vi "solar_cfg Simple.vi"(4 "Write If Not Found? (T)":bool=TRUE, 5 "Action (Read)":enum8{"Read", "Write"}(ring), 6 "Replace Existing Comments? (F)":bool, 7 "Section (\"\" = Filename)":string, 8 "error in (no error)":errorcluster, 10 "Key,Value,Comment":string[][](array[string]), 11 "Config Path (*.ini)":path) -> (0 "error out":errorcluster, 1 "Found?":bool, 2 "Values":string[](array[string]), 3 "dup Config Path":path)   [LabVIEW 2018]
doc: "This VI reads or writes a single item from a configuration file. The key is created if not found."
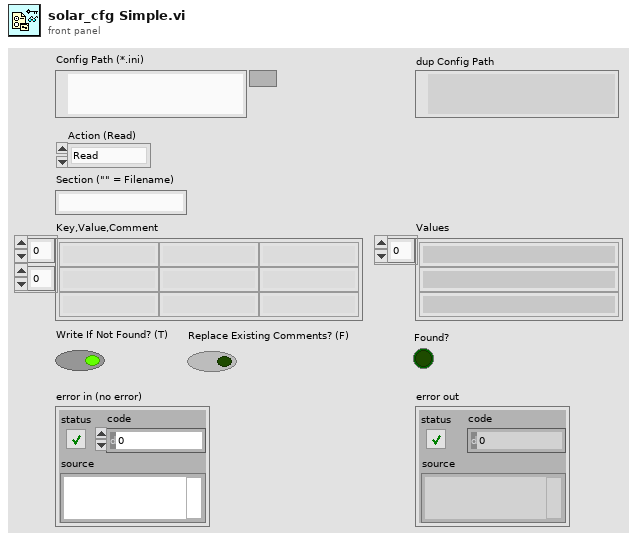
[diagram p1: front panel]
types:
  T1 = enum16{"open", "replace", "create", "open or create", "replace or create", "replace or create with confirmation"}
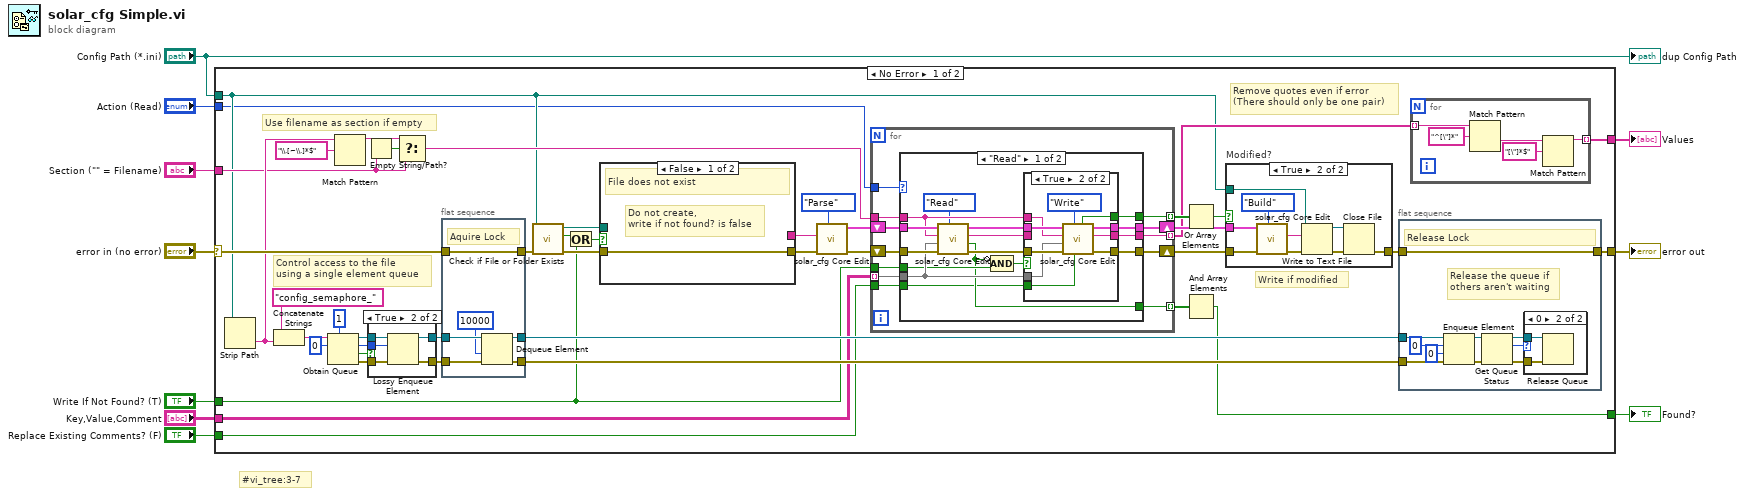
[diagram p0: block diagram]
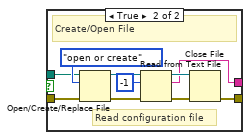
[diagram p2: hidden frame]
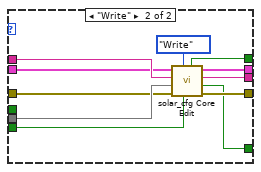
[diagram p4: hidden frame]
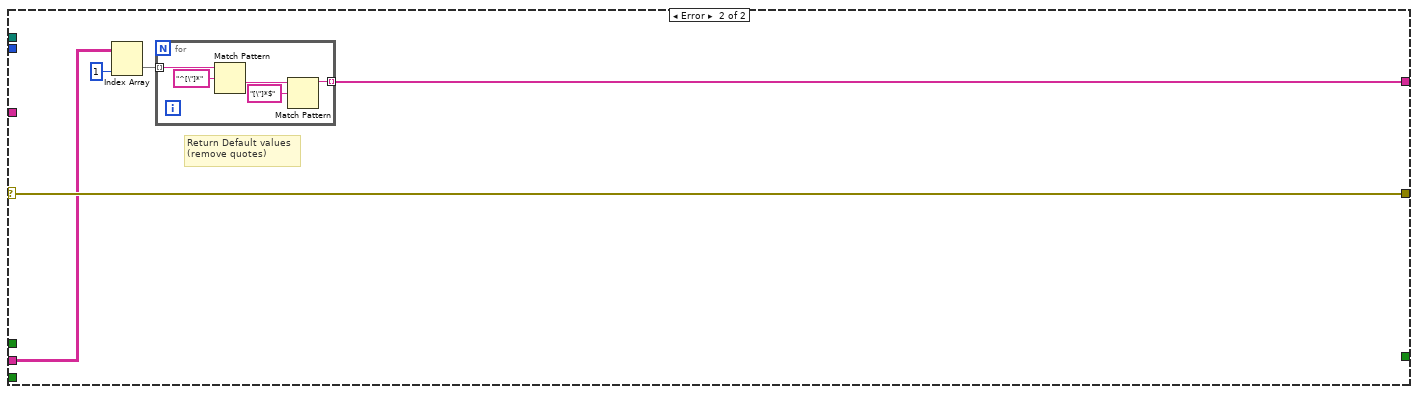
[diagram p8: hidden frame]
diagram:
  # "#vi_tree:3-7"
  n1 = case shown="No Error" "error in (no error)" {
    selector: "error in (no error)" -> [w42 w161]
    tunnel: "Action (Read)" -> [w14 _]
    tunnel: "Key,Value,Comment" -> [w23 w160]
    tunnel: "Config Path (*.ini)" -> [w16 _]
    tunnel: [w19 w157] -> w2
    tunnel: [w41 w161] -> w7
    tunnel: "Section (\"\" = Filename)" -> [w34 _]
    tunnel: "Write If Not Found? (T)" -> [w12 _]
    tunnel: [w22 _] -> w3
    tunnel: "Replace Existing Comments? (F)" -> [w18 _]
    frame No Error {
      w45 = u8 0
      # "Remove quotes even if error\n(There should only be one pair)"
      # "Use filename as section if empty"
      # "Write if modified"
      # "Control access to the file\nusing a single element queue"
      n2 = Strip Path(path=w16) -> (name=w37:string)  [unwired: 1 out]
      n3 = Concatenate Strings("config_semaphore_" ("string"), w37) -> (w47:string)
      n4 = Obtain Queue(max queue size (-1, unlimited)=1, name (unnamed)=w47, element data type=w45) -> (queue out=w50:refnum<queue>, created new?=w51:bool, error out=w49:errorcluster)  [unwired: 2 in]
      n5 = Match Pattern(string=w37, regular expression="\\.[~\\.]*$") -> (before substring=w35:string)  [unwired: 4 out]
      n6 = Empty String/Path?(string/path=w34) -> (empty?=w36:bool)
      n7 = case shown="True" w51 {
        tunnel: w50 -> [w141 w146]
        tunnel: w49 -> [w140 w145]
        tunnel: w45 -> [_ w144]
        tunnel: [w141 w143] -> w48
        tunnel: [w140 w142] -> w44
        frame False {
        }
        frame True {
          n8 = Lossy Enqueue Element(queue=w146, element=w144, error in (no error)=w145) -> (queue out=w143:refnum<queue>, error out=w142:errorcluster)  [unwired: 2 out]
        }
      }
      n9 = Select(t=w35, s=w36, f=w34) -> (s? t:f=w28:string)
      n10 = flat-sequence {
        tunnel: [w139] -> w53
        tunnel: w48 -> [w138]
        tunnel: w44 -> [w137]
        tunnel: [w135] -> w43
        tunnel: w42 -> [w135]
        tunnel: [w134] -> w39
        frame #0 {
          # "Aquire Lock"
          n11 = Dequeue Element(queue=w138, timeout in ms (-1)=10000, error in (no error)=w137) -> (queue out=w139:refnum<queue>, error out=w134:errorcluster)  [unwired: 2 out]
        }
      }
      n12 = call <vilib>:"Check if File or Folder Exists.vi"("error in (no error)"=w43, "path"=w16) -> ("error out"=w17:errorcluster, "file or folder exists?"=w13:bool, "dup path"=w15:path)  [unwired: 7 in]
      n13 = Or(x=w13, y=w12) -> (x .or. y?=w11:bool)
      n14 = case shown="False" w11 {
        tunnel: [w54 w58] -> w33
        tunnel: [_ w57] -> w32
        tunnel: w17 -> [w54 w56]
        tunnel: w15 -> [_ w55]
        frame False {
          # "Do not create,\nwrite if not found? is false"
          # "File does not exist"
        }
        frame True {
          # "Read configuration file"
          # "Create/Open File"
          n15 = Open/Create/Replace File(file path (use dialog)=w55, error in=w56, operation (0:open)=T1."open or create") -> (refnum out=w60:refnum<file>, error out=w61:errorcluster)  [unwired: 3 in, 1 out]
          n16 = Read from Text File(file (use dialog)=w60, count=-1, error in=w61) -> (refnum out=w63:refnum<file>, text=w57:string, error out=w64:errorcluster)  [unwired: 1 in, 1 out]
          n17 = Close File(refnum=w63, error in=w64) -> (error out=w58:errorcluster)  [unwired: 1 out]
        }
      }
      n18 = call "solar_cfg Core Edit.vi"("Action (Read)"=enum8{"Read", "Write", "Parse", "Build"}."Parse", "error in (no error)"=w33, "Section/String in"=w32) -> ("error out"=w30:errorcluster, "Sections out"=w29:cluster{"Section":string, "kvc":string[][]}[])  [unwired: 4 in, 3 out]
      n19 = for {
        tunnel: [w77] -> w26 mode=indexing
        tunnel: w14 -> [w72]
        tunnel: w23 -> [w71] mode=indexing
        shift-right: [w78] -> w27
        shift-left: w30 -> [w81]
        tunnel: w28 -> [w79]
        tunnel: [w75] -> w20 mode=indexing
        tunnel: w12 -> [w74]
        tunnel: [w73] -> w24 mode=indexing
        shift-right: [w76] -> w25
        shift-left: w29 -> [w80]
        tunnel: w18 -> [w70]
        n20 = case shown="\"Read\"" w72 {
          tunnel: w81 -> [w97 w113]
          tunnel: w80 -> [w96 w114]
          tunnel: w79 -> [w95 w121]
          tunnel: [w94 w120] -> w78
          tunnel: [w93 w119] -> w77
          tunnel: [w87 w118] -> w76
          tunnel: [w86 w117] -> w75
          tunnel: w71 -> [w85 w116]
          tunnel: w74 -> [w84 _]
          tunnel: [w83 w112] -> w73
          tunnel: w70 -> [w82 w111]
          frame "Read" {
            n21 = call "solar_cfg Core Edit.vi"("Action (Read)"=enum8{"Read", "Write", "Parse", "Build"}."Read", "error in (no error)"=w97, "kvc in"=w85, "Section/String in"=w95, "Sections in"=w96) -> ("error out"=w89:errorcluster, "Found?"=w83:bool, "Value/String out"=w88:string, "Sections out"=w92:cluster{"Section":string, "kvc":string[][]}[])  [unwired: 2 in, 1 out]
            n22 = Compound Arithmetic op=AND(invert w83, w84) -> (w91:bool)
            n23 = case "Not Found & Create?" shown="True" w91 {
              tunnel: w92 -> [w98 w110]
              tunnel: w89 -> [w100 w107]
              tunnel: [w100 w106] -> w94
              tunnel: w95 -> [_ w109]
              tunnel: w85 -> [_ w105]
              tunnel: w88 -> [w99 _]
              tunnel: [w99 w104] -> w86
              tunnel: [w98 w103] -> w87
              tunnel: [_ w102] -> w93
              tunnel: w82 -> [_ w101]
              frame False {
              }
              frame True {
                # "Create Key"
                n24 = call "solar_cfg Core Edit.vi"("Write Comments? (T)"=w101, "Action (Read)"=enum8{"Read", "Write", "Parse", "Build"}."Write", "error in (no error)"=w107, "kvc in"=w105, "Section/String in"=w109, "Sections in"=w110) -> ("error out"=w106:errorcluster, "Value/String out"=w104:string, "Sections out"=w103:cluster{"Section":string, "kvc":string[][]}[], "Dirty?"=w102:bool)  [unwired: 1 in, 1 out]
              }
            }
          }
          frame "Write" {
            n25 = call "solar_cfg Core Edit.vi"("Write Comments? (T)"=w111, "Action (Read)"=enum8{"Read", "Write", "Parse", "Build"}."Write", "error in (no error)"=w113, "kvc in"=w116, "Section/String in"=w121, "Sections in"=w114) -> ("error out"=w120:errorcluster, "Found?"=w112:bool, "Value/String out"=w117:string, "Sections out"=w118:cluster{"Section":string, "kvc":string[][]}[], "Dirty?"=w119:bool)  [unwired: 1 in]
          }
        }
      }
      n26 = Or Array Elements(Boolean array=w26) -> (logical OR=w21:bool)
      n27 = And Array Elements(Boolean array=w24) -> (logical AND=w22:bool)
      n28 = case "Modified?" shown="True" w21 {
        tunnel: [w147 w155] -> w40
        tunnel: w27 -> [w147 w151]
        tunnel: w16 -> [_ w153]
        tunnel: w25 -> [_ w149]
        frame False {
        }
        frame True {
          n29 = call "solar_cfg Core Edit.vi"("Action (Read)"=enum8{"Read", "Write", "Parse", "Build"}."Build", "error in (no error)"=w151, "Sections in"=w149) -> ("error out"=w150:errorcluster, "Value/String out"=w148:string)  [unwired: 4 in, 3 out]
          n30 = Write to Text File(file (use dialog)=w153, text=w148, error in=w150) -> (refnum out=w154:refnum<file>, error out=w156:errorcluster)  [unwired: 1 in, 1 out]
          n31 = Close File(refnum=w154, error in=w156) -> (error out=w155:errorcluster)  [unwired: 1 out]
        }
      }
      n32 = flat-sequence {
        tunnel: w53 -> [w131]
        tunnel: [w128] -> w41
        tunnel: w40 -> [w128]
        tunnel: w39 -> [w127]
        frame #0 {
          # "Release the queue if\nothers aren't waiting"
          # "Release Lock"
          n33 = Enqueue Element(queue=w131, element=u8 0, timeout in ms (-1)=0, error in (no error)=w127) -> (queue out=w123:refnum<queue>, error out=w122:errorcluster)  [unwired: 1 out]
          n34 = Get Queue Status(queue=w123, error in (no error)=w122) -> (queue out=w125:refnum<queue>, # pending remove=w124:i32, error out=w126:errorcluster)  [unwired: 1 in, 5 out]
          n35 = case shown="0" w124 {
            tunnel: w125 -> [_ w133]
            tunnel: w126 -> [_ w132]
            frame Default {
            }
            frame 0 {
              n36 = Release Queue(queue=w133, error in (no error)=w132) -> ()  [unwired: 1 in, 3 out]
            }
          }
        }
      }
      n37 = for {
        tunnel: w20 -> [w66] mode=indexing
        tunnel: [w65] -> w19 mode=indexing
        n38 = Match Pattern(string=w66, regular expression="^[\"]*") -> (after substring=w67:string)  [unwired: 1 in, 3 out]
        n39 = Match Pattern(string=w67, regular expression="[\"]*$") -> (before substring=w65:string)  [unwired: 1 in, 3 out]
      }
    }
    frame Error {
      # "Return Default values\n(remove quotes)"
      n40 = Index Array(array=w160, index (col)=1 ("disabled index (col)")) -> (element=w158:string[])  [unwired: 1 in]
      n41 = for {
        tunnel: w158 -> [w163] mode=indexing
        tunnel: [w162] -> w157 mode=indexing
        n42 = Match Pattern(string=w163, regular expression="^[\"]*") -> (after substring=w164:string)  [unwired: 1 in, 3 out]
        n43 = Match Pattern(string=w164, regular expression="[\"]*$") -> (before substring=w162:string)  [unwired: 1 in, 3 out]
      }
    }
  }
  "error out" <- w7
  "Found?" <- w3
  "Values" <- w2
  "dup Config Path" <- "Config Path (*.ini)"
